vi "MyOwn PID Encoders.vi"(9 "Current Input":dbl, 10 "Wanted End":dbl) -> (3 "Output":dbl)   [LabVIEW 2017]
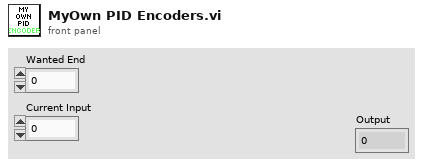
[diagram p1: front panel]
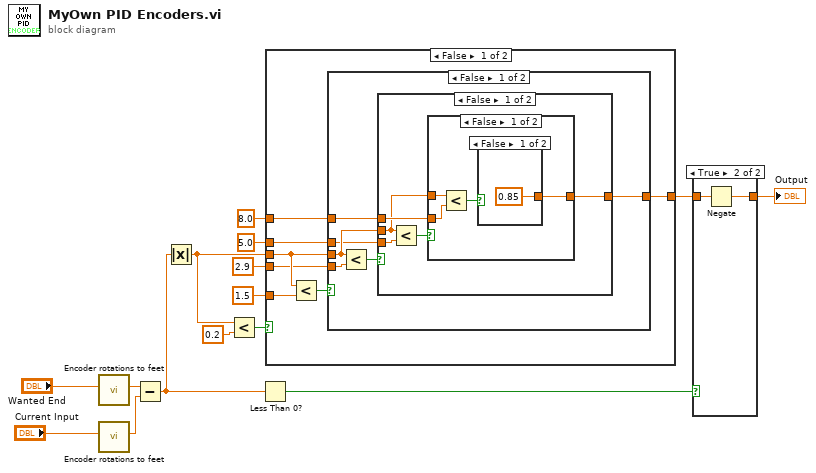
[diagram p0: block diagram]
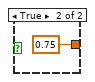
[diagram p3: hidden frame]
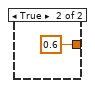
[diagram p4: hidden frame]
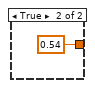
[diagram p5: hidden frame]
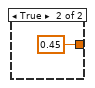
[diagram p6: hidden frame]
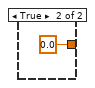
[diagram p7: hidden frame]
diagram:
  n1 = call "Encoder rotations to feet.vi"("Encoder Rotations"="Wanted End") -> ("Feet"=w15:dbl)  [unwired: 10 in]
  n2 = call "Encoder rotations to feet.vi"("Encoder Rotations"="Current Input") -> ("Feet"=w14:dbl)  [unwired: 10 in]
  n3 = Subtract(x=w15, y=w14) -> (x-y=w5:dbl)
  n4 = Absolute Value(x=w5) -> (abs(x)=w6:dbl)
  n5 = Less?(x=w6, y=0.2) -> (x < y?=w13:bool)
  n6 = Less Than 0?(x=w5) -> (x < 0?=w9:bool)
  n7 = case shown="False" w13 {
    tunnel: w6 -> [w19 _]
    tunnel: [w20 0.0] -> w8
    tunnel: 1.5 -> [w22 _]
    tunnel: 2.9 -> [w18 _]
    tunnel: 8.0 -> [w17 _]
    tunnel: 5.0 -> [w16 _]
    frame False {
      n8 = Less?(x=w19, y=w22) -> (x < y?=w21:bool)
      n9 = case shown="False" w21 {
        tunnel: [w27 0.45] -> w20
        tunnel: w19 -> [w25 _]
        tunnel: w18 -> [w28 _]
        tunnel: w17 -> [w24 _]
        tunnel: w16 -> [w23 _]
        frame False {
          n10 = Less?(x=w25, y=w28) -> (x < y?=w26:bool)
          n11 = case shown="False" w26 {
            tunnel: [w33 0.54] -> w27
            tunnel: w25 -> [w30 _]
            tunnel: w24 -> [w32 _]
            tunnel: w23 -> [w29 _]
            frame False {
              n12 = Less?(x=w30, y=w29) -> (x < y?=w31:bool)
              n13 = case shown="False" w31 {
                tunnel: [w36 0.6] -> w33
                tunnel: w30 -> [w34 _]
                tunnel: w32 -> [w35 _]
                frame False {
                  n14 = Less?(x=w34, y=w35) -> (x < y?=w37:bool)
                  n15 = case shown="False" w37 {
                    tunnel: [0.85 0.75] -> w36
                    frame False {
                    }
                    frame True {
                    }
                  }
                }
                frame True {
                }
              }
            }
            frame True {
            }
          }
        }
        frame True {
        }
      }
    }
    frame True {
    }
  }
  n16 = case shown="True" w9 {
    tunnel: w8 -> [w44 w46]
    tunnel: [w44 w45] -> w7
    frame False {
    }
    frame True {
      n17 = Negate(x=w46) -> (-x=w45:dbl)
    }
  }
  "Output" <- w7
